vi "API_LoadTiffImage.vi"(6 "Timeout (ms)":u32, 7 "Wait (F)":bool, 8 "error in (no error)":errorcluster, 10 "PathToImage":path, 11 "DLP2 in":refnum<class "DLP2.lvclass">) -> (0 "error out":errorcluster, 2 "ImageData":T1, 3 "DLP2 out":refnum<class "DLP2.lvclass">)   [LabVIEW 2022 SP3, in "DLP2.lvclass"]
doc: "Developed by Kevin Thompson\nkevin@thompsonengineering.net\n\nCopyright 2018\nThompson Engineering, LLC"
uses:
  DLP2.lvclass
  DataTypes/AsynCmd_Temp01--enum.ctl
  DLP2.lvclass/DLP2.ctl
  TopLevel/Typedefs/TiffImageData--Cluster.ctl
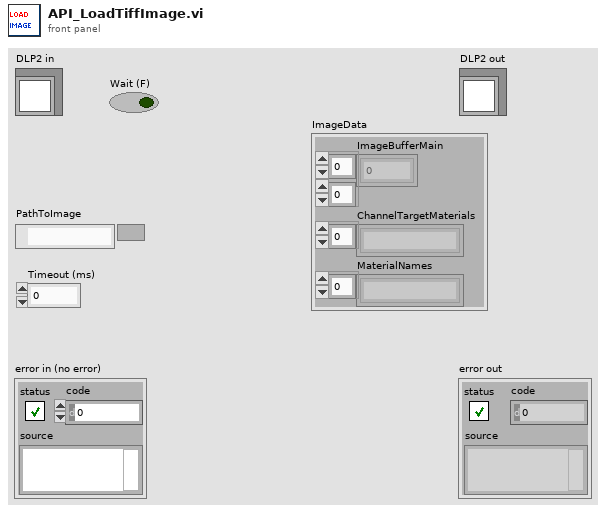
[diagram p1: front panel]
types:
  T1 = typedef "TiffImageData--Cluster.ctl" = cluster{"ImageBufferMain":u8[][], "ChannelTargetMaterials":string[], "MaterialNames":string[]}
  T2 = typedef "DLP2.lvclass/AsynCmd_Temp01--enum.ctl" = enum16{"LoadTiffImage"}
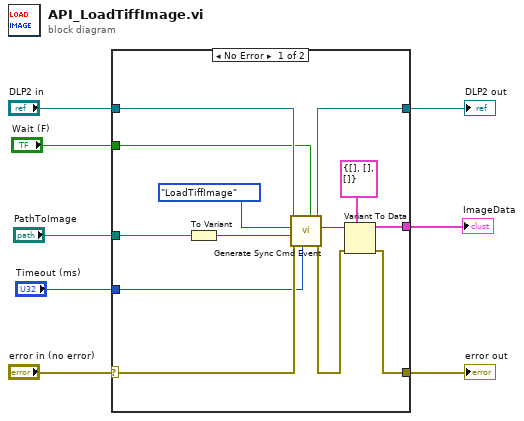
[diagram p0: block diagram]
diagram:
  n1 = case shown="No Error" "error in (no error)" {
    selector: "error in (no error)" -> [w19 w23]
    tunnel: [w11 w23] -> w7
    tunnel: [w20 w22] -> w5
    tunnel: "DLP2 in" -> [w21 w22]
    tunnel: "PathToImage" -> [w17 _]
    tunnel: "Wait (F)" -> [w15 _]
    tunnel: "Timeout (ms)" -> [w14 _]
    tunnel: [w9 _] -> w1
    frame No Error {
      n2 = To Variant(anything=w17) -> (Variant=w16:variant)
      n3 = call "Generate Sync Cmd Event.vi"("Wait (F)"=w15, "Timeout (ms)"=w14, "error in (no error)"=w19, "vData"=w16, "AsyncCmd"=AsynCmd_Temp01--enum."LoadTiffImage", "DLP2 in"=w21) -> ("error out"=w12:errorcluster, "Return Value"=w13:variant, "DLP2 out"=w20:refnum<class "DLP2.lvclass">)  [unwired: 3 in]
      n4 = Variant To Data(error in=w12, type=T1 {"ImageBufferMain"=[], "ChannelTargetMaterials"=[], "MaterialNames"=[]} ("ImageData"), Variant=w13) -> (data=w9:T1, error out=w11:errorcluster)
    }
    frame Error {
    }
  }
  "error out" <- w7
  "DLP2 out" <- w5
  "ImageData" <- w1
